vi "Initialize Modbus Client TCP.vi"(5 "timeout, ms (300)":u32=300, 7 "protocol (TCP)":enum16{"RTU", "ASCII", "TCP"}(ring)=enum."TCP", 8 "error in (no error)":errorcluster, 9 "station address (255)":u8=255, 10 "port (502)":u16=502, 11 "ip address":string) -> (0 "error out":errorcluster, 3 "MODBUS Out":refnum<class "Modbus.lvclass">)   [LabVIEW 2020, in "Library Instrument & Equipement.lvlib" / "Library Relay_Board.lvlib" / "Modbus.lvclass"]
doc: "Initializes TCP connection to Modbus server using specified settings."
uses:
  Modbus.lvclass
  Modbus.lvclass/Modbus.ctl
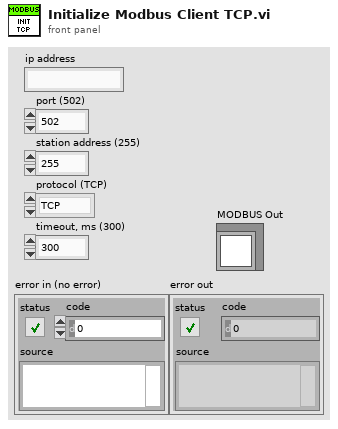
[diagram p1: front panel]
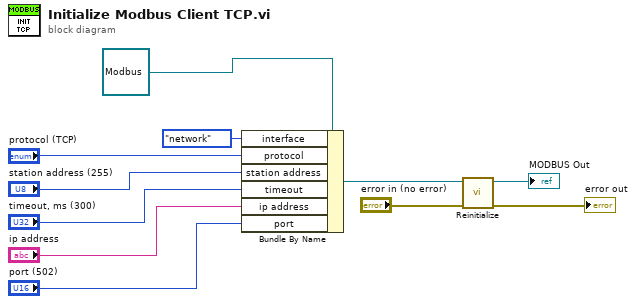
[diagram p0: block diagram]
diagram:
  n1 = Bundle By Name(cluster=refnum<class "Modbus.lvclass"> refnum ("MODBUS in"), "interface"=enum16{"serial", "network"}."network", "protocol"="protocol (TCP)", "station address"="station address (255)", "timeout"="timeout, ms (300)", "ip address"="ip address", "port"="port (502)") -> (w10:refnum<class "Modbus.lvclass">)
  n2 = call "Reinitialize.vi"("error in (no error)"="error in (no error)", "MODBUS in"=w10) -> ("error out"=→"error out":errorcluster, "MODBUS Out"=→"MODBUS Out":refnum<class "Modbus.lvclass">)  [unwired: 8 in]
